vi "Data Logger Global.vi"(0 "WebDAV Push":bool, 1 "In Spec":bool[](array[boolean])=[FALSE, FALSE, FALSE, FALSE, FALSE, FALSE], 2 "Current Step":i32=2, 3 "Step Time Left":dbl=0.21101045608520508, 4 "Pump Data":T2={"Voltages"=[0.015201568603515625, 0.00335693359375, 0.003021240234375, 0.12260055541992188, 0.06085968017578125, 0.052234649658203125], "PumpCurrent"=[0.015201568603515625, 0.00335693359375, 0.003021240234375, 0.12260055541992188, 0.06085968017578125, 0.052234649658203125], "Speed"=[0.0, 0.0, 0.0, 0.0, 0.0, 0.0], "ControllerCurrent"=[0.015201568603515625, 0.00335693359375, 0.003021240234375, 0.12260055541992188, 0.06085968017578125, 0.052234649658203125], "Pressure"=[0.015201568603515625, 0.00335693359375, 0.003021240234375, 0.12260055541992188, 0.06085968017578125, 0.052234649658203125], "Flow"=[0.0, 0.0, 0.0, 0.125, 0.0625, 0.0625], "Elapsed Time:"=[7.1, 7.1, 7.1, 458133.45, 458138.85000000003, 458126.75], "Avg Pressure"=0.0, "Avg Speed"=0.0} {"Elapsed Time:" format="%<%H:%M:%S>t"; "Speed" format="%#_4f"; "ControllerCurrent" format="%#.1g"; "Pressure" format="%#.0f"; "Flow" format="%#.0f"; "PumpCurrent" format="%#.1g"; "Voltages" format="%#.0f"}, 5 "Tank Data":T1 {"PS Actual (V):" format="%.2f"; "Temp1" format="%#_2g"; "Temp2" format="%#_2g"}, 8 "Write (F)":bool) -> (14 "WebDAV Push OUT":bool, 15 "In Spec OUT":bool[](array[boolean]), 16 "Current Step OUT":i32, 17 "Step Time Left OUT":dbl, 18 "Pump Data OUT":T2={"Voltages"=[0.0, 0.05908203125, 0.06982421875, 0.05908203125, 0.06982421875, 0.0859375], "PumpCurrent"=[0.0015967955457961394, 0.0015950073791676203, 0.0015981739242389562, 0.0015920643549248493, 0.001590499709124895, 0.0015808510600251774], "Speed"=[0.0, 0.0, 0.0, 0.0, 0.0, 0.0], "ControllerCurrent"=[0.0, 0.0, 0.0, 0.0, 0.0, 0.0], "Pressure"=[0.0, 0.0, 0.0, 0.0, 0.0, 0.0], "Flow"=[0.0, 0.0, 0.0, 0.0, 0.0, 0.0], "Elapsed Time:"=[4074.9003000000002, 4074.9003000000002, 4074.9003000000002, 4074.9003000000002, 4074.9003000000002, 4074.9003000000002], "Avg Pressure"=0.0, "Avg Speed"=0.0} {"Elapsed Time:" format="%<%H:%M:%S>t"; "Speed" format="%#_4f"; "ControllerCurrent" format="%#.1g"; "Pressure" format="%#.0f"; "Flow" format="%#.0f"; "PumpCurrent" format="%#.1g"; "Voltages" format="%#.0f"}, 19 "Tank Data OUT":T1 {"PS Actual (V):" format="%.2f"; "Temp1" format="%#_2g"; "Temp2" format="%#_2g"})   [LabVIEW 2013]
uses:
  Controls/Pump Data.ctl
  Controls/Tank Data.ctl
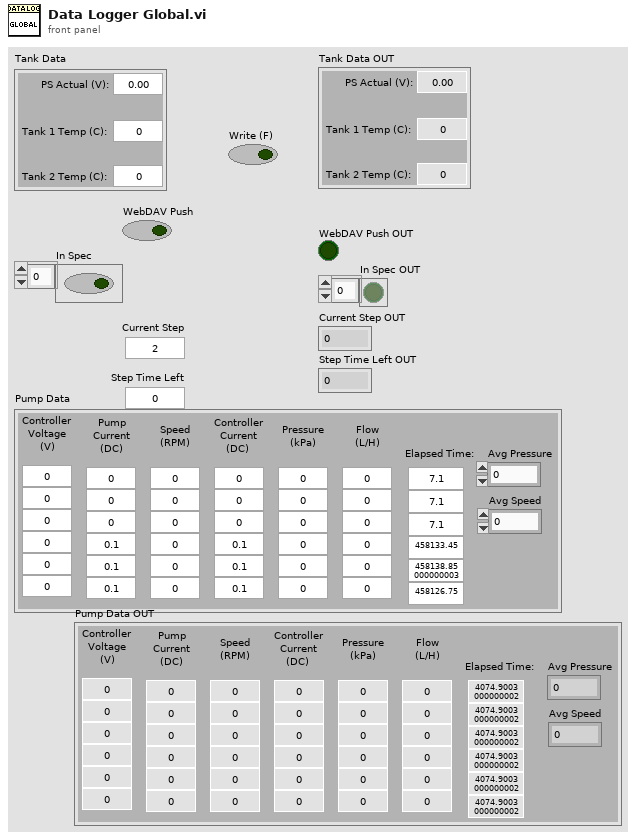
[diagram p1: front panel]
types:
  T1 = typedef "Tank Data.ctl" = cluster{"PS Actual (V):":dbl, "Temp1":dbl, "Temp2":dbl}
  T2 = typedef "Pump Data.ctl" = cluster{"Voltages":dbl[], "PumpCurrent":dbl[], "Speed":dbl[], "ControllerCurrent":dbl[], "Pressure":dbl[], "Flow":dbl[], "Elapsed Time:":dbl[], "Avg Pressure":dbl, "Avg Speed":dbl}
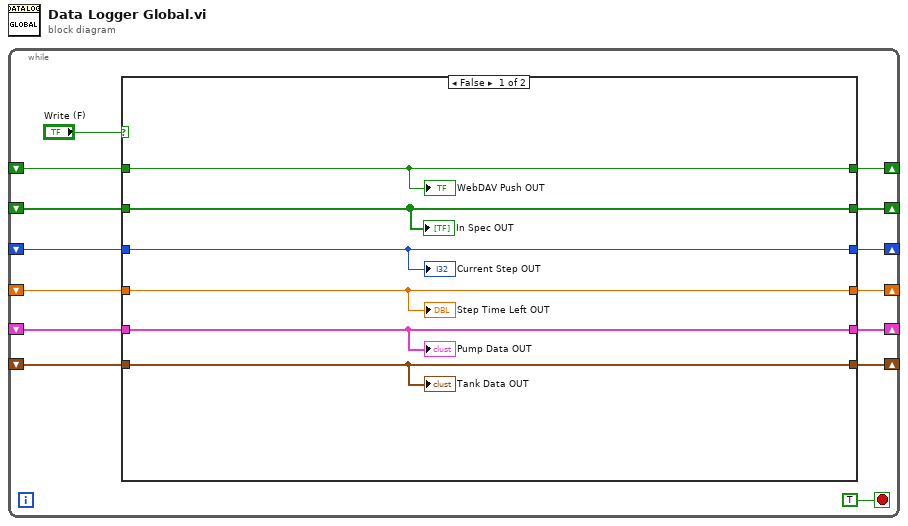
[diagram p0: block diagram]
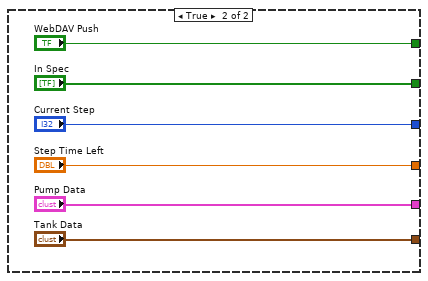
[diagram p2: hidden frame]
diagram:
  n1 = while {
    shift-right: [w12] -> _
    shift-left: _ -> [w9]
    shift-right: [w11] -> _
    shift-left: _ -> [w8]
    shift-right: [w10] -> _
    shift-left: _ -> [w7]
    shift-right: [w6] -> _
    shift-left: _ -> [w4]
    shift-right: [w5] -> _
    shift-left: _ -> [w3]
    shift-right: [w2] -> _
    shift-left: _ -> [w1]
    stop <- TRUE stop-if-true
    n2 = case shown="False" "Write (F)" {
      tunnel: [w20 "WebDAV Push"] -> w12
      tunnel: [w19 "Current Step"] -> w11
      tunnel: [w18 "Step Time Left"] -> w10
      tunnel: w9 -> [w20 _]
      tunnel: w8 -> [w19 _]
      tunnel: w7 -> [w18 _]
      tunnel: [w17 "Pump Data"] -> w6
      tunnel: [w16 "Tank Data"] -> w5
      tunnel: w4 -> [w17 _]
      tunnel: w3 -> [w16 _]
      tunnel: [w15 "In Spec"] -> w2
      tunnel: w1 -> [w15 _]
      frame False {
        "WebDAV Push OUT" <- w20
        "Current Step OUT" <- w19
        "Step Time Left OUT" <- w18
        "Pump Data OUT" <- w17
        "Tank Data OUT" <- w16
        "In Spec OUT" <- w15
      }
      frame True {
      }
    }
  }
